vi "Station-Run.vi"(8 "error in (no error)":errorcluster) -> (0 "error out":errorcluster)   [LabVIEW 2016]
uses:
  Station.Action.ctl
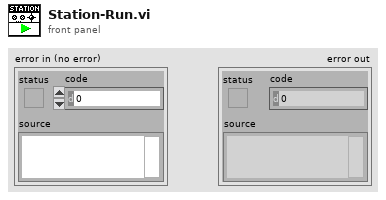
[diagram p1: front panel]
types:
  T1 = typedef "Station.Action.ctl" = enum32{"idle", "constructor", "destructor", "--- Station ---", "Hardware.Init", "Status.Update", "Status.Clear", "Order", "Init", "Ready", "Start", "Run", "Stop", "Error", "Home", "Done", "Seq.Run", "Seq.Done", "Tower.Update", "Mode.Select", "Emg", "Emg.Reset", "Emg.Check", "Home.Check", "Prod.Check", "Butt.Check"}
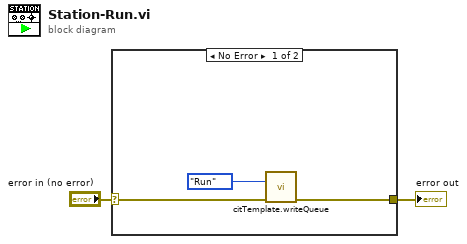
[diagram p0: block diagram]
diagram:
  n1 = case shown="No Error" "error in (no error)" {
    selector: "error in (no error)" -> [w3 w6]
    tunnel: [w5 w6] -> w2
    frame No Error {
      n2 = call "citTemplate.writeQueue.vi"("event in (if not connected:all statemachine with data event)"=Station.Action."Run" ("Action"), "error in (no error)"=w3) -> ("error out"=w5:errorcluster)  [unwired: 13 in]
    }
    frame Error {
    }
  }
  "error out" <- w2
